vi "Find steep and swap.vi"(11 "Line":T1) -> (2 "steep":bool, 3 "Line Out":T1)   [LabVIEW 2019]
uses:
  TypeDefs/Line.ctl
  TypeDefs/Pixel.ctl
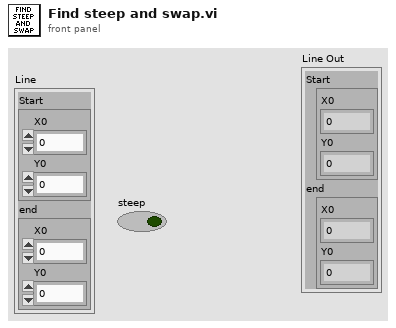
[diagram p1: front panel]
types:
  T1 = typedef "Line.ctl" = cluster{"Start":T2, "end":T2}
  T2 = typedef "Pixel.ctl" = cluster{"X0":i16, "Y0":i16}
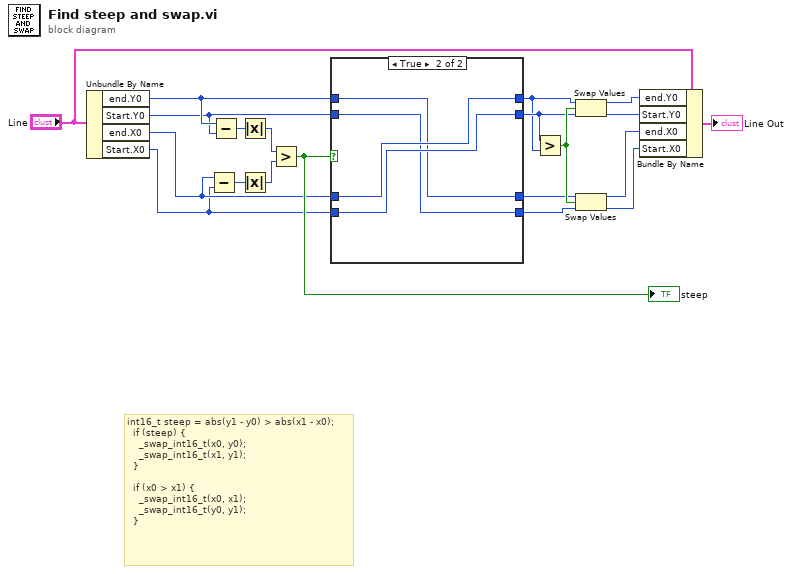
[diagram p0: block diagram]
diagram:
  # "int16_t steep = abs(y1 - y0) > abs(x1 - x0);\n  if (steep) {\n    _swap_int16_t(x0, y0);\n    _swap_int16_t(x1, y1);\n  }\n\n  if (x0 > x1) {\n    _swap_int16_t(x0, x1);\n    _swap_int16_t(y0, y1);\n  }"
  n1 = Unbundle By Name("Line") -> ("end.Y0"=w10:i16, "Start.Y0"=w9:i16, "end.X0"=w8:i16, "Start.X0"=w7:i16)
  n2 = Subtract(x=w8, y=w7) -> (x-y=w19:i16)
  n3 = Subtract(x=w10, y=w9) -> (x-y=w18:i16)
  n4 = Absolute Value(x=w18) -> (abs(x)=w20:i16)
  n5 = Absolute Value(x=w19) -> (abs(x)=w11:i16)
  n6 = Greater?(x=w20, y=w11) -> (0:w17:bool)
  "steep" <- w17
  n7 = case shown="True" w17 {
    tunnel: w9 -> [w24 w26]
    tunnel: w10 -> [w21 w25]
    tunnel: w7 -> [w23 w28]
    tunnel: w8 -> [w22 w27]
    tunnel: [w24 w28] -> w13
    tunnel: [w21 w27] -> w12
    tunnel: [w23 w26] -> w15
    tunnel: [w22 w25] -> w14
    frame False {
    }
    frame True {
    }
  }
  n8 = Greater?(x=w13, y=w12) -> (0:w16:bool)
  n9 = Swap Values(12:w12, 13:w16, 14:w13) -> (1:w5:i16, 3:w4:i16)
  n10 = Swap Values(12:w14, 13:w16, 14:w15) -> (1:w3:i16, 3:w2:i16)
  n11 = Bundle By Name(cluster="Line", "end.Y0"=w5, "Start.Y0"=w4, "end.X0"=w3, "Start.X0"=w2) -> (→"Line Out":T1)
